vi "Recieve Response with Result.vi"(4 "Finished":bool=TRUE, 6 "Result":refnum<class "Mag Lab Result.lvclass">, 8 "error in (no error)":errorcluster, 9 "Requestor":string, 10 "Requestee":string, 11 "RUS Measurement in":refnum<class "RUS Measurement.lvclass">) -> (0 "error out":errorcluster, 3 "RUS Measurement out":refnum<class "RUS Measurement.lvclass">)   [LabVIEW 2015, in "RUS Measurement.lvclass"]
uses:
  RUS Measurement.lvclass
  Mag Lab Result/Mag Lab Result.lvclass
  <vilib>/ActorFramework/Actor/Actor.lvclass/Actor.ctl
  Mag Lab Root Messages/Recieve Request for Result Msg/Recieve Request for Result Msg.lvclass/Recieve Request for Result Msg.ctl
  <vilib>/ActorFramework/Message Enqueuer/Message Enqueuer.lvclass/Message Enqueuer.ctl
  RUS Measurement.lvclass/RUS Measurement.ctl
  Mag Lab Result/Mag Lab Result.lvclass/Mag Lab Result.ctl
  Mag Lab Measure Base Messages/Select Graph Channels Msg/Select Graph Channels Msg.lvclass/Select Graph Channels Msg.ctl
  RUS Parameters.ctl
  Mag Lab Root/Mag Lab Root.lvclass/Mag Lab Root.ctl
  Mag Lab Result/Find Peaks Result/Find Peaks Result.lvclass
  Mag Lab Root Messages/Recieve Response with Result Msg/Recieve Response with Result Msg.lvclass/Recieve Response with Result Msg.ctl
  Mag Lab Result/Read Group Name.vi
  Read Sweep chunk.vi
  Write Sweep chunk.vi
  Mag Lab Root/Read Name.vi
  Mag Lab Root/Read Original requestor.vi
  Write Active.vi
  Mag Lab Root/Read Request time.vi
  Mag Lab Result/Write Sets pace.vi
  Mag Lab Result/Write Result time.vi
  Mag Lab Result/Write Group Name.vi
  Mag Lab Result/Write Name.vi
  <vilib>/ActorFramework/Message Enqueuer/Enqueue.vi
  <vilib>/ActorFramework/Message Priority Queue/Priority Enqueue.vi
  Mag Lab Root Messages/Recieve Request for Result Msg/Recieve Request for Result Msg.lvclass
  Mag Lab Measure Base Messages/Select Graph Channels Msg/Select Graph Channels Msg.lvclass
  Mag Lab Properties/Mag Lab Parameters.lvclass
  Mag Lab Root Messages/Recieve Response with Result Msg/Recieve Response with Result Msg.lvclass
  <vilib>/ActorFramework/Actor/Actor.lvclass
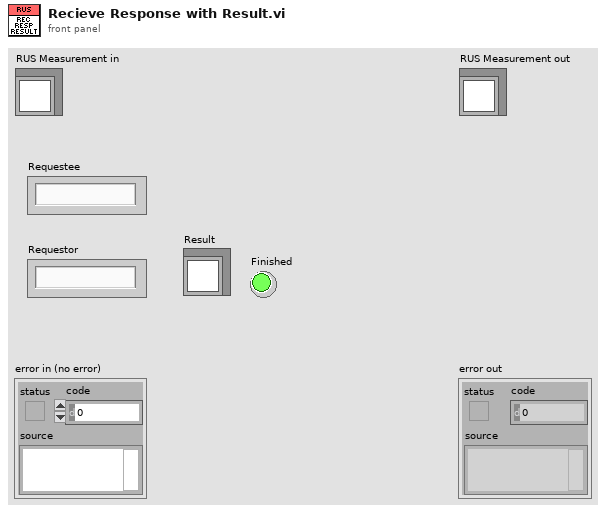
[diagram p1: front panel]
types:
  T1 = typedef "RUS Parameters.ctl" = cluster{"Start frequency":dbl, "End frequency":dbl, "Duration":dbl, "Averaging":dbl, "Find peaks":bool}
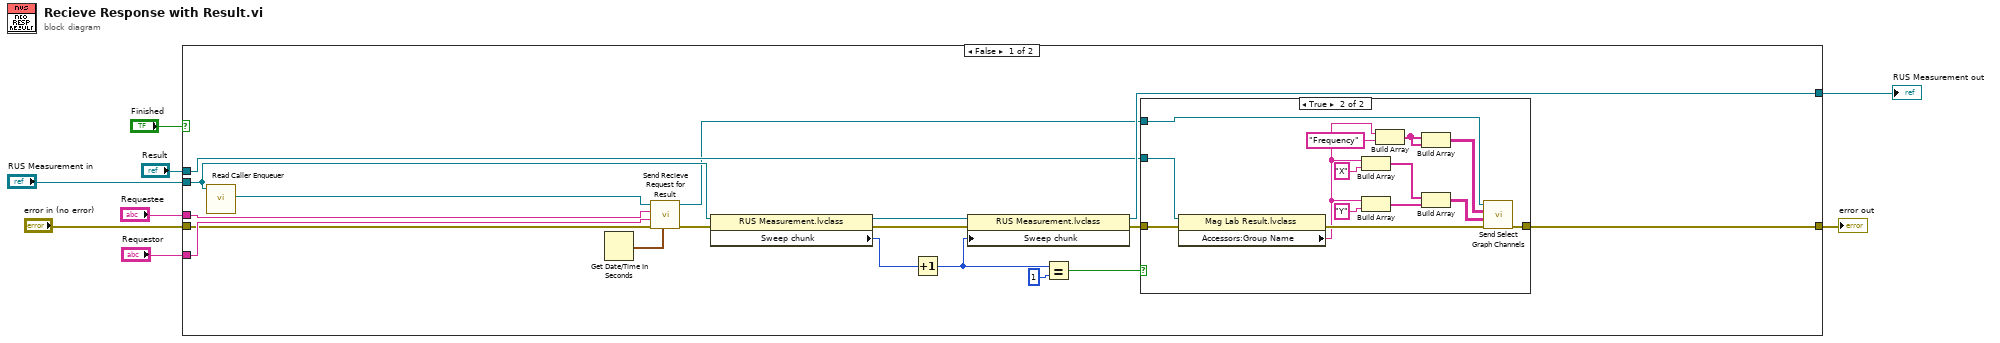
[diagram p0: block diagram]
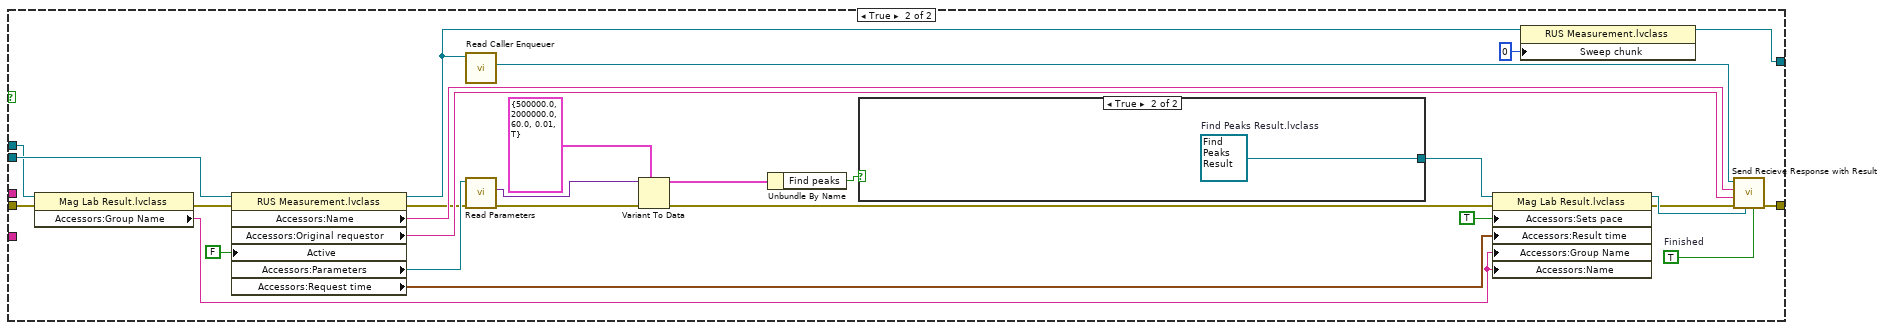
[diagram p3: hidden frame]
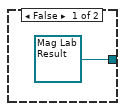
[diagram p4: hidden frame]
diagram:
  n1 = case shown="False" "Finished" {
    tunnel: "RUS Measurement in" -> [w21 w64]
    tunnel: "Requestee" -> [w25 _]
    tunnel: "Requestor" -> [w24 _]
    tunnel: "error in (no error)" -> [w22 w54]
    tunnel: [w15 w65] -> w4
    tunnel: [w19 w43] -> w2
    tunnel: "Result" -> [w17 w57]
    frame False {
      n2 = call <vilib>:"Read Caller Enqueuer.vi"("Actor"=w21) -> ("Caller Enqueuer"=w26:refnum<class "Message Enqueuer.lvclass">)  [unwired: 10 in]
      n3 = Get Date/Time In Seconds() -> (seconds since 1Jan1904=w23:timestamp)
      n4 = call "Send Recieve Request for Result.vi"("Request time"=w23, "error in (no error)"=w22, "Requestor"=w24, "Requestee"=w25, "Message Enqueuer"=w26) -> ("error out"=w12:errorcluster, "Message Enqueuer out"=w16:refnum<class "Message Enqueuer.lvclass">)  [unwired: 5 in]
      n5 = property class="RUS Measurement.lvclass"(reference=w21, error in=w12) -> (reference out=w20:refnum<class "RUS Measurement.lvclass">, error out=w13:errorcluster, "Sweep chunk"=w18:i32)
      n6 = Increment(x=w18) -> (x+1=w11:i32)
      n7 = property class="RUS Measurement.lvclass"(reference=w20, error in=w13, "Sweep chunk"=w11) -> (reference out=w19:refnum<class "RUS Measurement.lvclass">, error out=w14:errorcluster)
      n8 = Equal?(x=w11, y=1) -> (x = y?=w9:bool)
      n9 = case shown="True" w9 {
        tunnel: w17 -> [_ w41]
        tunnel: w16 -> [_ w40]
        tunnel: [w27 w37] -> w15
        tunnel: w14 -> [w27 w36]
        frame False {
        }
        frame True {
          n10 = property class="Mag Lab Result.lvclass"(reference=w41, error in=w36) -> (error out=w35:errorcluster, "Accessors:Group Name"=w31:string)  [unwired: 1 out]
          n11 = Build Array(w31, "X" ("String")) -> (w28:string[])
          n12 = Build Array(w31, "Y" ("String")) -> (w30:string[])
          n13 = Build Array(w31, "Frequency" ("String")) -> (w29:string[])
          n14 = Build Array(w29, w29) -> (w39:string[][])
          n15 = Build Array(w28, w30) -> (w38:string[][])
          n16 = call "Send Select Graph Channels.vi"("error in (no error)"=w35, "Y Group Channels"=w38, "X Group Channels"=w39, "Message Enqueuer"=w40) -> ("error out"=w37:errorcluster)  [unwired: 6 in, 1 out]
        }
      }
    }
    frame True {
      w63 = TRUE  # Finished
      n17 = property class="Mag Lab Result.lvclass"(reference=w57, error in=w54) -> (error out=w53:errorcluster, "Accessors:Group Name"=w52:string)  [unwired: 1 out]
      n18 = property class="RUS Measurement.lvclass"(reference=w64, error in=w53, "Active"=FALSE) -> (reference out=w67:refnum<class "RUS Measurement.lvclass">, error out=w50:errorcluster, "Accessors:Name"=w58:string, "Accessors:Original requestor"=w66:string, "Accessors:Parameters"=w51:refnum<class "Mag Lab Parameters.lvclass">, "Accessors:Request time"=w55:timestamp)
      n19 = call <vilib>:"Read Caller Enqueuer.vi"("Actor"=w67) -> ("Caller Enqueuer"=w68:refnum<class "Message Enqueuer.lvclass">)  [unwired: 10 in]
      n20 = call-dynamic "Read Parameters.vi"("error in (no error)"=w50, "Mag Lab Parameters in"=w51) -> ("error out"=w49:errorcluster, "Parameters"=w48:variant)  [unwired: 7 in, 1 out]
      n21 = Variant To Data(error in=w49, type=T1 {"Start frequency"=500000.0, "End frequency"=2000000.0, "Duration"=60.0, "Averaging"=0.01, "Find peaks"=TRUE} ("Parameters"), Variant=w48) -> (data=w46:T1, error out=w45:errorcluster)
      n22 = Unbundle By Name(w46) -> ("Find peaks"=w44:bool)
      n23 = case shown="True" w44 {
        tunnel: [refnum<class "Mag Lab Result.lvclass"> refnum ("Mag Lab Result.lvclass") w70] -> w56
        frame False {
        }
        frame True {
          w70 = refnum<class "Find Peaks Result.lvclass"> refnum  # Find Peaks Result.lvclass
        }
      }
      n24 = property class="Mag Lab Result.lvclass"(reference=w56, error in=w45, "Accessors:Sets pace"=TRUE ("Sets pace"), "Accessors:Result time"=w55, "Accessors:Group Name"=w52, "Accessors:Name"=w52) -> (reference out=w62:refnum<class "Mag Lab Result.lvclass">, error out=w60:errorcluster)
      n25 = property class="RUS Measurement.lvclass"(reference=w67, "Sweep chunk"=0) -> (reference out=w43:refnum<class "RUS Measurement.lvclass">)  [unwired: 1 in, 1 out]
      n26 = call "Send Recieve Response with Result.vi"("Finished"=w63, "Result"=w62, "error in (no error)"=w60, "Requestor"=w66, "Requestee"=w58, "Message Enqueuer"=w68) -> ("error out"=w65:errorcluster)  [unwired: 4 in, 1 out]
    }
  }
  "error out" <- w4
  "RUS Measurement out" <- w2
